vi "Car Wash.vi"() -> ()   [LabVIEW 2021]
uses:
  Customized control/Wash Controller.ctl
panel:
  out "Timer":dbl
  in  "Stop Button":bool
  in  "Air Dry\nPosition\nSwitch":bool
  in  "Main Wash\nPosition\nSwitch":bool
  in  "Under Body \nWash Position\nSwitch":bool
  out "Vehicle Out of Position":bool
  out "Air Dry":bool
  out "Clear Water Rinse":bool
  out "Main High Pressure Wash":bool
  out "Soap Application":bool
  out "Under Body Wash":bool
  in  "Economy Wash":bool
  in  "Deluxe Wash":bool
  # "Car Wash Controller System"
  # "Timer"
  # "Car Wash Simulation Switches"
  # "Car Wash Indicators"
  # "Purchase Selection"
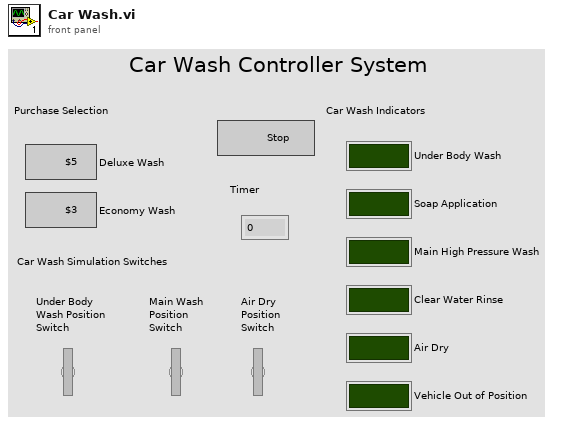
[diagram p1: front panel]
types:
  T1 = typedef "Wash Controller.ctl" = enum16{"Initialization", "Operation mode", "Deluxe wash", "Economy wash", "End"}
  T2 = enum8{"Enabled", "Disabled", "Disabled and Grayed Out"}
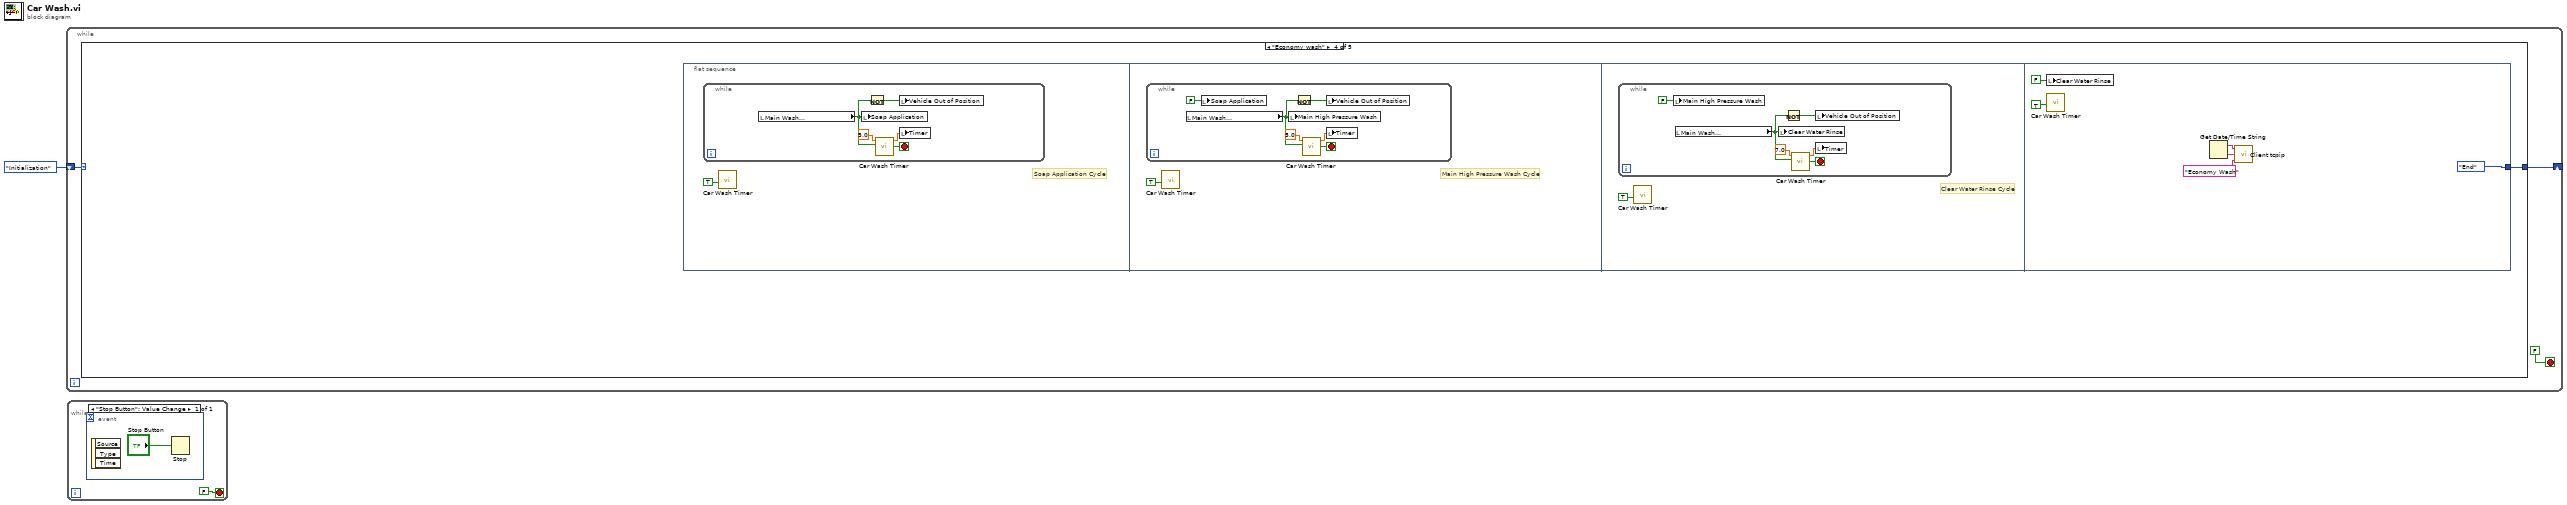
[diagram p0: block diagram]
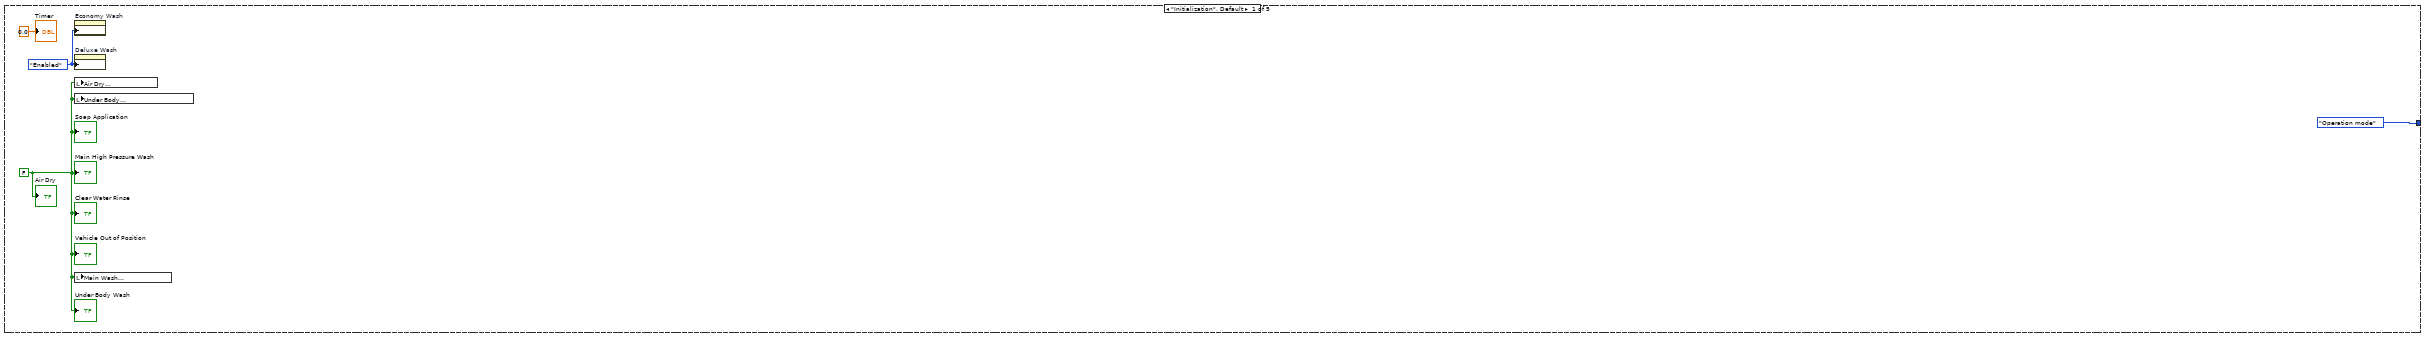
[diagram p2: hidden frame]
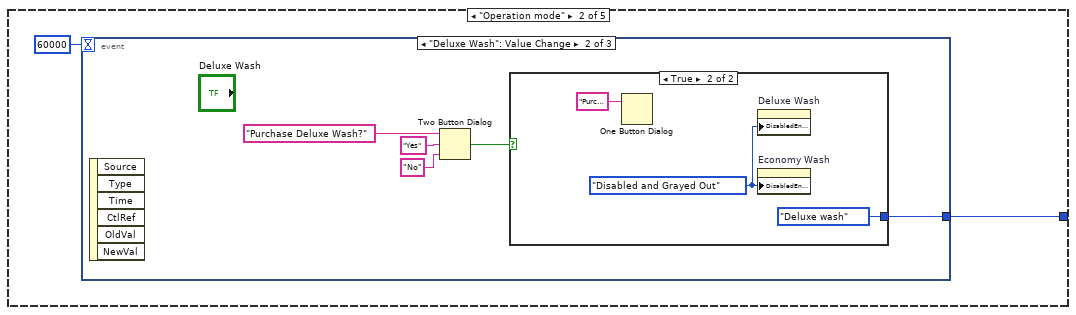
[diagram p3: hidden frame]
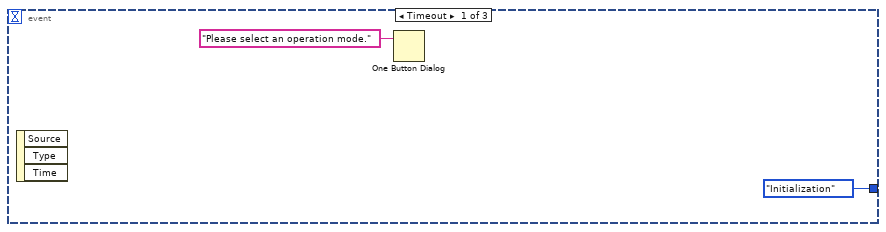
[diagram p4: hidden frame]
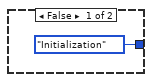
[diagram p5: hidden frame]
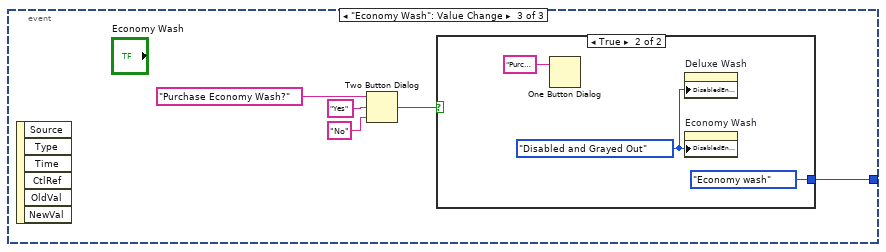
[diagram p6: hidden frame]
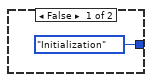
[diagram p7: hidden frame]
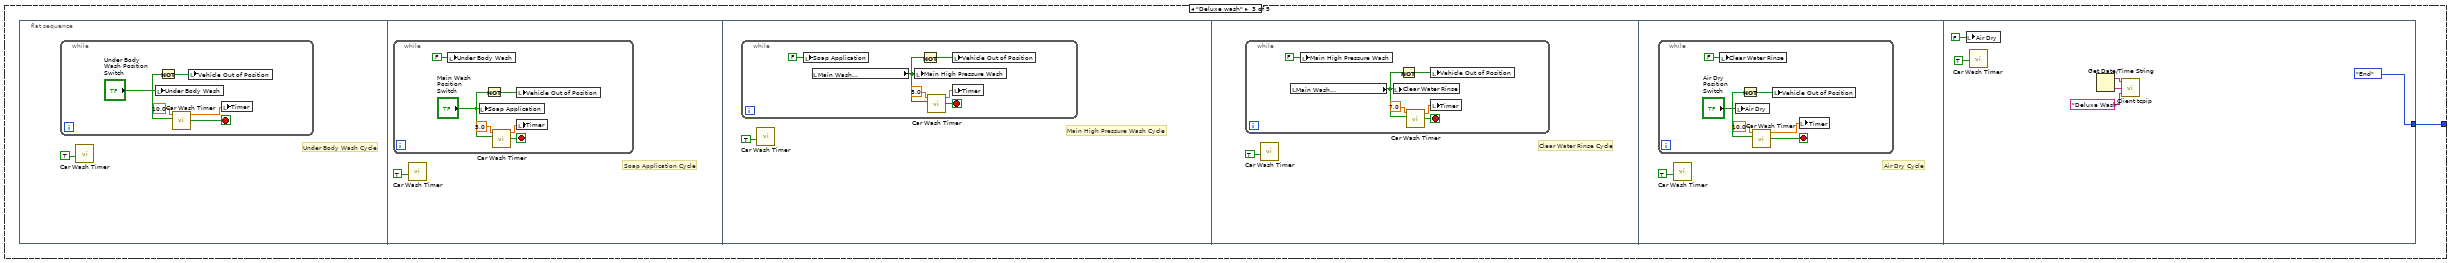
[diagram p8: hidden frame]
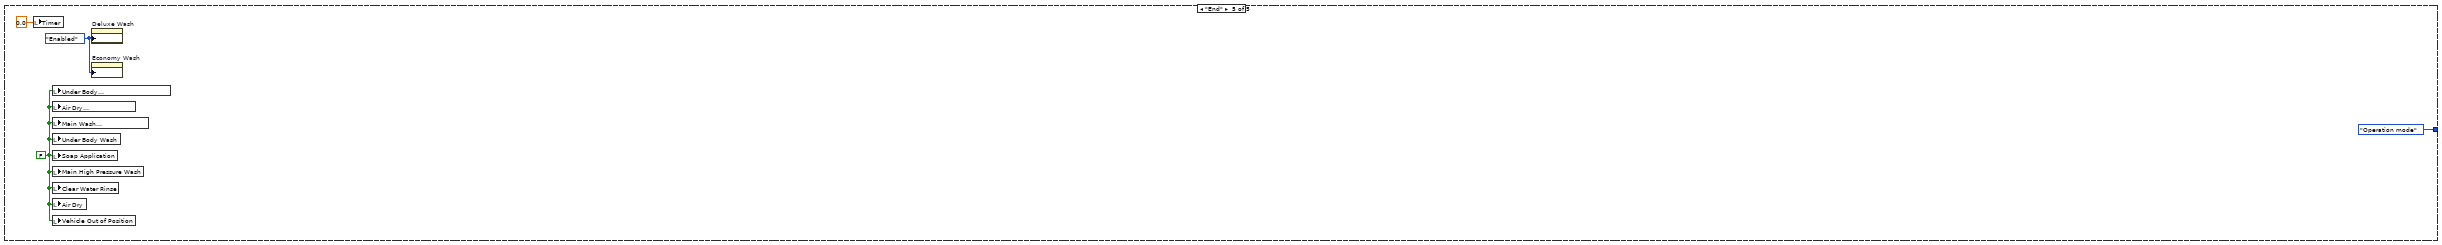
[diagram p9: hidden frame]
diagram:
  n1 = while {
    shift-right: [w2] -> _
    shift-left: Wash_Controller."Initialization" -> [w4]
    stop <- FALSE stop-if-true
    n2 = case shown="\"Economy wash\"" w4 {
      tunnel: [Wash_Controller."Operation mode" w10 w31 w72 Wash_Controller."Operation mode"] -> w2
      frame "Initialization", Default {
        w7 = T2."Enabled" ("Disabled")
        w6 = FALSE ("Under Body Wash")
        n3 = property on="Economy Wash" class="Bool"("DisabledEnum"=w7) -> ()  [unwired: 2 in, 2 out]
        n4 = property on="Deluxe Wash" class="Bool"("DisabledEnum"=w7) -> ()  [unwired: 2 in, 2 out]
        n5 = local write "Air Dry\nPosition\nSwitch"(w6) -> ()
        n6 = local write "Under Body \nWash Position\nSwitch"(w6) -> ()
        n7 = local write "Main Wash\nPosition\nSwitch"(w6) -> ()
        "Under Body Wash" <- w6
        "Soap Application" <- w6
        "Main High Pressure Wash" <- w6
        "Clear Water Rinse" <- w6
        "Air Dry" <- w6
        "Vehicle Out of Position" <- w6
        "Timer" <- 0.0 ("Timer")
      }
      frame "Operation mode" {
        n8 = event shown="[1] \"Deluxe Wash\": Value Change" {
          selector: _ -> [_ _ _]
          dyn-events: _ -> [_ _ _]
          timeout: 60000 -> [_ _ _]
          tunnel: [Wash_Controller."Initialization" w13 w22] -> w10
          event Timeout {
            n9 = event-data() -> ()  [unwired: 1 in, 3 out]
            n10 = One Button Dialog(message="Please select an operation mode.") -> ()  [unwired: 1 in, 1 out]
          }
          event "Deluxe Wash": Value Change {
            n11 = event-data() -> ()  [unwired: 1 in, 6 out]
            n12 = Two Button Dialog(message="Purchase Deluxe Wash?", 1:"No" ("T button name (\"OK\")"), 2:"Yes" ("T button name (\"OK\")")) -> (T button?=w14:bool)
            n13 = case shown="True" w14 {
              tunnel: [Wash_Controller."Initialization" Wash_Controller."Deluxe wash"] -> w13
              frame False {
              }
              frame True {
                w21 = T2."Disabled and Grayed Out" ("Disabled")
                n14 = One Button Dialog(message="Purchase Successful. Please move your vehicle to the underwash section.") -> ()  [unwired: 1 in, 1 out]
                n15 = property on="Deluxe Wash" class="Bool"("DisabledEnum"=w21) -> ()  [unwired: 2 in, 2 out]
                n16 = property on="Economy Wash" class="Bool"("DisabledEnum"=w21) -> ()  [unwired: 2 in, 2 out]
              }
            }
          }
          event "Economy Wash": Value Change {
            n17 = event-data() -> ()  [unwired: 1 in, 6 out]
            n18 = Two Button Dialog(message="Purchase Economy Wash?", 1:"No" ("F button name (\"Cancel\")"), 2:"Yes" ("T button name (\"OK\")")) -> (T button?=w23:bool)
            n19 = case shown="True" w23 {
              tunnel: [Wash_Controller."Initialization" Wash_Controller."Economy wash"] -> w22
              frame False {
              }
              frame True {
                w30 = T2."Disabled and Grayed Out" ("Disabled")
                n20 = One Button Dialog(message="Purchase Successful. Please move your vehicle to the main wash section.\n") -> ()  [unwired: 1 in, 1 out]
                n21 = property on="Deluxe Wash" class="Bool"("DisabledEnum"=w30) -> ()  [unwired: 2 in, 2 out]
                n22 = property on="Economy Wash" class="Bool"("DisabledEnum"=w30) -> ()  [unwired: 2 in, 2 out]
              }
            }
          }
        }
      }
      frame "Deluxe wash" {
        n23 = flat-sequence {
          tunnel: [Wash_Controller."End"] -> w31
          frame #0 {
            # "Under Body Wash Cycle"
            n24 = while {
              stop <- w34 stop-if-true
              n25 = local write "Under Body Wash"("Under Body \nWash Position\nSwitch") -> ()
              n26 = Not(x="Under Body \nWash Position\nSwitch") -> (.not. x?=w33:bool)
              n27 = call "Car Wash Timer.vi"("Controller"="Under Body \nWash Position\nSwitch", "Time"=10.0) -> ("Elapsed"=w34:bool, "Elapsed Time"=w35:dbl)  [unwired: 2 in, 1 out]
              n28 = local write "Vehicle Out of Position"(w33) -> ()
              n29 = local write "Timer"(w35) -> ()
            }
            n30 = call "Car Wash Timer.vi"("Reset"=TRUE) -> ()  [unwired: 3 in, 3 out]
          }
          frame #1 {
            # "Soap Application Cycle"
            n31 = while {
              stop <- w43 stop-if-true
              n32 = local write "Under Body Wash"(FALSE ("Under Body Wash")) -> ()
              n33 = local write "Soap Application"("Main Wash\nPosition\nSwitch") -> ()
              n34 = Not(x="Main Wash\nPosition\nSwitch") -> (.not. x?=w39:bool)
              n35 = call "Car Wash Timer.vi"("Controller"="Main Wash\nPosition\nSwitch", "Time"=5.0) -> ("Elapsed"=w43:bool, "Elapsed Time"=w42:dbl)  [unwired: 2 in, 1 out]
              n36 = local write "Vehicle Out of Position"(w39) -> ()
              n37 = local write "Timer"(w42) -> ()
            }
            n38 = call "Car Wash Timer.vi"("Reset"=TRUE) -> ()  [unwired: 3 in, 3 out]
          }
          frame #2 {
            # "Main High Pressure Wash Cycle"
            n39 = while {
              stop <- w47 stop-if-true
              n40 = local write "Soap Application"(FALSE ("Soap Application")) -> ()
              n41 = local read "Main Wash\nPosition\nSwitch"() -> (w50:bool)
              n42 = local write "Main High Pressure Wash"(w50) -> ()
              n43 = Not(x=w50) -> (.not. x?=w46:bool)
              n44 = call "Car Wash Timer.vi"("Controller"=w50, "Time"=5.0) -> ("Elapsed"=w47:bool, "Elapsed Time"=w51:dbl)  [unwired: 2 in, 1 out]
              n45 = local write "Vehicle Out of Position"(w46) -> ()
              n46 = local write "Timer"(w51) -> ()
            }
            n47 = call "Car Wash Timer.vi"("Reset"=TRUE) -> ()  [unwired: 3 in, 3 out]
          }
          frame #3 {
            # "Clear Water Rinse Cycle"
            n48 = while {
              stop <- w54 stop-if-true
              n49 = local read "Main Wash\nPosition\nSwitch"() -> (w56:bool)
              n50 = local write "Main High Pressure Wash"(FALSE ("Main High Pressure Wash")) -> ()
              n51 = local write "Clear Water Rinse"(w56) -> ()
              n52 = Not(x=w56) -> (.not. x?=w53:bool)
              n53 = call "Car Wash Timer.vi"("Controller"=w56, "Time"=7.0) -> ("Elapsed"=w54:bool, "Elapsed Time"=w57:dbl)  [unwired: 2 in, 1 out]
              n54 = local write "Vehicle Out of Position"(w53) -> ()
              n55 = local write "Timer"(w57) -> ()
            }
            n56 = call "Car Wash Timer.vi"("Reset"=TRUE) -> ()  [unwired: 3 in, 3 out]
          }
          frame #4 {
            # "Air Dry Cycle"
            n57 = while {
              stop <- w63 stop-if-true
              n58 = local write "Clear Water Rinse"(FALSE ("Clear Water Rinse")) -> ()
              n59 = local write "Air Dry"("Air Dry\nPosition\nSwitch") -> ()
              n60 = Not(x="Air Dry\nPosition\nSwitch") -> (.not. x?=w60:bool)
              n61 = call "Car Wash Timer.vi"("Controller"="Air Dry\nPosition\nSwitch", "Time"=10.0) -> ("Elapsed"=w63:bool, "Elapsed Time"=w64:dbl)  [unwired: 2 in, 1 out]
              n62 = local write "Vehicle Out of Position"(w60) -> ()
              n63 = local write "Timer"(w64) -> ()
            }
            n64 = call "Car Wash Timer.vi"("Reset"=TRUE) -> ()  [unwired: 3 in, 3 out]
          }
          frame #5 {
            n65 = local write "Air Dry"(FALSE ("Air Dry")) -> ()
            n66 = call "Car Wash Timer.vi"("Reset"=TRUE) -> ()  [unwired: 3 in, 3 out]
            n67 = Get Date/Time String() -> (date string=w68:string, time string=w67:string)  [unwired: 3 in]
            n68 = call "Client tcpip.vi"("Type of wash"="Deluxe Wash", "Time"=w67, "Date"=w68) -> ()
          }
        }
      }
      frame "Economy wash" {
        n69 = flat-sequence {
          tunnel: [Wash_Controller."End"] -> w72
          frame #0 {
            # "Soap Application Cycle"
            n70 = while {
              stop <- w77 stop-if-true
              n71 = local read "Main Wash\nPosition\nSwitch"() -> (w75:bool)
              n72 = local write "Soap Application"(w75) -> ()
              n73 = Not(x=w75) -> (.not. x?=w74:bool)
              n74 = call "Car Wash Timer.vi"("Controller"=w75, "Time"=5.0) -> ("Elapsed"=w77:bool, "Elapsed Time"=w76:dbl)  [unwired: 2 in, 1 out]
              n75 = local write "Vehicle Out of Position"(w74) -> ()
              n76 = local write "Timer"(w76) -> ()
            }
            n77 = call "Car Wash Timer.vi"("Reset"=TRUE) -> ()  [unwired: 3 in, 3 out]
          }
          frame #1 {
            # "Main High Pressure Wash Cycle"
            n78 = while {
              stop <- w81 stop-if-true
              n79 = local read "Main Wash\nPosition\nSwitch"() -> (w84:bool)
              n80 = local write "Soap Application"(FALSE ("Soap Application")) -> ()
              n81 = local write "Main High Pressure Wash"(w84) -> ()
              n82 = Not(x=w84) -> (.not. x?=w80:bool)
              n83 = call "Car Wash Timer.vi"("Controller"=w84, "Time"=5.0) -> ("Elapsed"=w81:bool, "Elapsed Time"=w85:dbl)  [unwired: 2 in, 1 out]
              n84 = local write "Vehicle Out of Position"(w80) -> ()
              n85 = local write "Timer"(w85) -> ()
            }
            n86 = call "Car Wash Timer.vi"("Reset"=TRUE) -> ()  [unwired: 3 in, 3 out]
          }
          frame #2 {
            # "Clear Water Rinse Cycle"
            n87 = while {
              stop <- w88 stop-if-true
              n88 = local write "Main High Pressure Wash"(FALSE ("Main High Pressure Wash")) -> ()
              n89 = local read "Main Wash\nPosition\nSwitch"() -> (w90:bool)
              n90 = local write "Clear Water Rinse"(w90) -> ()
              n91 = Not(x=w90) -> (.not. x?=w87:bool)
              n92 = call "Car Wash Timer.vi"("Controller"=w90, "Time"=7.0) -> ("Elapsed"=w88:bool, "Elapsed Time"=w91:dbl)  [unwired: 2 in, 1 out]
              n93 = local write "Vehicle Out of Position"(w87) -> ()
              n94 = local write "Timer"(w91) -> ()
            }
            n95 = call "Car Wash Timer.vi"("Reset"=TRUE) -> ()  [unwired: 3 in, 3 out]
          }
          frame #3 {
            n96 = local write "Clear Water Rinse"(FALSE ("Clear Water Rinse")) -> ()
            n97 = call "Car Wash Timer.vi"("Reset"=TRUE) -> ()  [unwired: 3 in, 3 out]
            n98 = Get Date/Time String() -> (date string=w95:string, time string=w94:string)  [unwired: 3 in]
            n99 = call "Client tcpip.vi"("Type of wash"="Economy Wash", "Time"=w94, "Date"=w95) -> ()
          }
        }
      }
      frame "End" {
        w100 = T2."Enabled" ("Disabled")
        w101 = FALSE ("Under Body \nWash Position\nSwitch")
        n100 = local write "Timer"(0.0 ("Timer")) -> ()
        n101 = local write "Under Body \nWash Position\nSwitch"(w101) -> ()
        n102 = local write "Air Dry\nPosition\nSwitch"(w101) -> ()
        n103 = local write "Main Wash\nPosition\nSwitch"(w101) -> ()
        n104 = local write "Under Body Wash"(w101) -> ()
        n105 = local write "Soap Application"(w101) -> ()
        n106 = local write "Main High Pressure Wash"(w101) -> ()
        n107 = local write "Clear Water Rinse"(w101) -> ()
        n108 = local write "Air Dry"(w101) -> ()
        n109 = local write "Vehicle Out of Position"(w101) -> ()
        n110 = property on="Deluxe Wash" class="Bool"("DisabledEnum"=w100) -> ()  [unwired: 2 in, 2 out]
        n111 = property on="Economy Wash" class="Bool"("DisabledEnum"=w100) -> ()  [unwired: 2 in, 2 out]
      }
    }
  }
  n112 = while {
    stop <- FALSE stop-if-true
    n113 = event shown="[0] \"Stop Button\": Value Change" {
      selector: _ -> [_]
      dyn-events: _ -> [_]
      timeout: _ -> [_]
      event "Stop Button": Value Change {
        n114 = event-data() -> ()  [unwired: 1 in, 3 out]
        n115 = Stop(stop? (T)="Stop Button") -> ()
      }
    }
  }
